vi "Add Data Set to Statistics.vi"(10 "JSON Data Set":refnum<class "JSON Value.lvclass">, 11 "Statistics in":refnum<class "JSON Value.lvclass">) -> (3 "Statistics":refnum<class "JSON Value.lvclass">)   [LabVIEW 2020, in "Library Commun.lvlib" / "JSON Statistics.lvclass"]
uses:
  JSON Statistics.lvclass
  JSON Value/JSON Value.lvclass
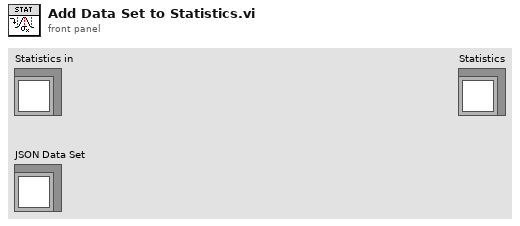
[diagram p1: front panel]
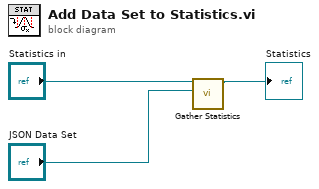
[diagram p0: block diagram]
diagram:
  n1 = call-dynamic "Gather Statistics.vi"("JSON Value"="JSON Data Set", "Statistics in"="Statistics in") -> ("Statistics out"=→"Statistics":refnum<class "JSON Value.lvclass">)  [unwired: 9 in]
